vi "Set Intensity Graph Z Range.vi"(8 "error in (no error)":errorcluster, 9 "Maximum [1]":dbl=1.0, 10 "Minimum [0]":dbl, 11 "graph_utilities in":refnum<class "graph_utilities.lvclass">) -> (0 "error out":errorcluster, 3 "graph_utilities out":refnum<class "graph_utilities.lvclass">)   [LabVIEW 2020, in "graph_utilities.lvclass"]
doc: "Set the Z scale range <b>Minimum</b> and <b>Maximum</b> values."
uses:
  graph_utilities.lvclass
  graph_utilities.lvclass/graph_utilities.ctl
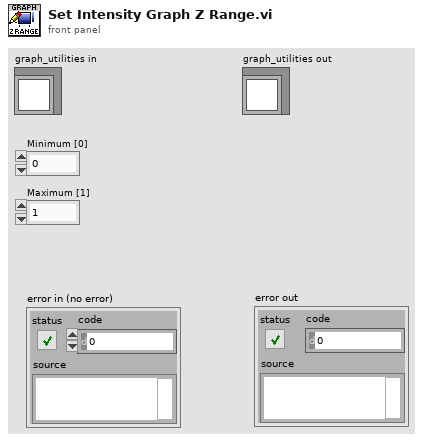
[diagram p1: front panel]
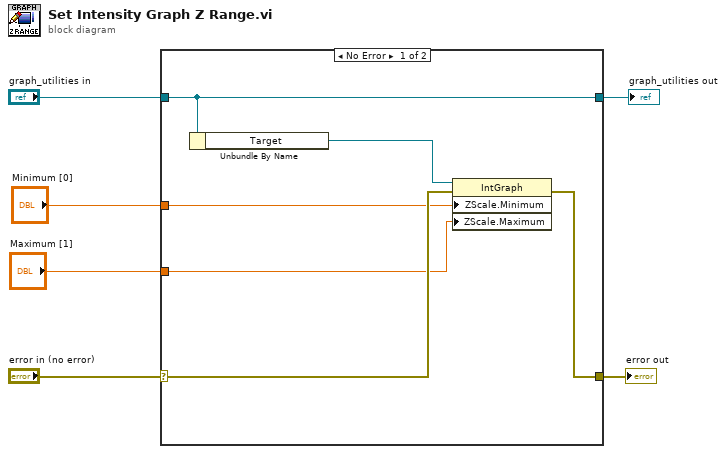
[diagram p0: block diagram]
diagram:
  n1 = case shown="No Error" "error in (no error)" {
    selector: "error in (no error)" -> [w11 w14]
    tunnel: [w12 w14] -> w6
    tunnel: "graph_utilities in" -> [w10 w13]
    tunnel: [w10 w13] -> w3
    tunnel: "Minimum [0]" -> [w8 _]
    tunnel: "Maximum [1]" -> [w7 _]
    frame No Error {
      n2 = Unbundle By Name(w10) -> ("Target"=w9:refnum<vi>)
      n3 = property on="Property Node" class="IntGraph"(reference=w9, error in=w11, "ZScale.Minimum"=w8, "ZScale.Maximum"=w7) -> (error out=w12:errorcluster)  [unwired: 1 out]
    }
    frame Error {
    }
  }
  "error out" <- w6
  "graph_utilities out" <- w3
